vi "Set PortNumber.vi"(8 "error in (no error)":errorcluster, 10 "PortNumber":i32, 11 "SessionOptions in":refnum<class "SessionOptions.lvclass">) -> (0 "error out":errorcluster, 3 "SessionOptions out":refnum<class "SessionOptions.lvclass">)   [LabVIEW 2015, in "SessionOptions.lvclass"]
uses:
  SessionOptions.lvclass
  SessionOptions.lvclass/SessionOptions.ctl
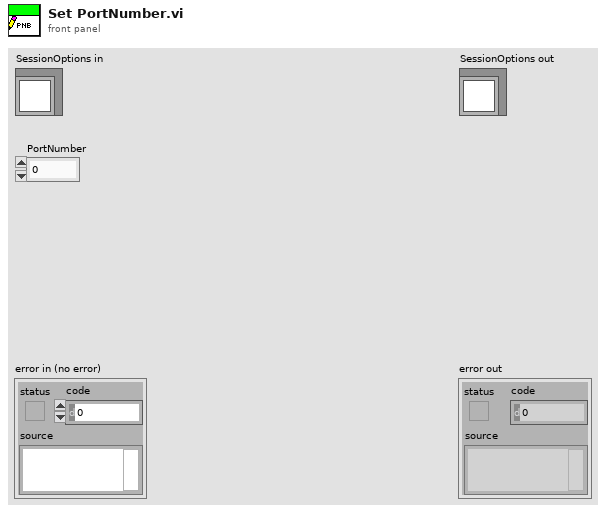
[diagram p1: front panel]
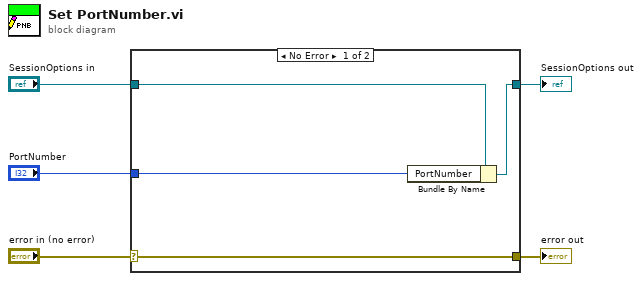
[diagram p0: block diagram]
diagram:
  n1 = case shown="No Error" "error in (no error)" {
    selector: "error in (no error)" -> [w9 w10]
    tunnel: [w9 w10] -> w4
    tunnel: [w7 w11] -> w2
    tunnel: "SessionOptions in" -> [w8 w11]
    tunnel: "PortNumber" -> [w6 _]
    frame No Error {
      n2 = Bundle By Name(cluster=w8, "PortNumber"=w6) -> (w7:refnum<class "SessionOptions.lvclass">)
    }
    frame Error {
    }
  }
  "error out" <- w4
  "SessionOptions out" <- w2
